vi "BlingLoop.vi"(5 "Cancel Ref":refnum<notifier>, 10 "Camera Ring Color":refnum<vi>, 11 "Target":string="10.24.68.5") -> (0 "error out":errorcluster)   [LabVIEW 2018]
uses:
  LedControlStates.ctl
  BlingLibrary/ControlState.ctl
  BlingLibrary/ConnectionType.ctl
  BlingLibrary/UdpConnection.ctl
  BlingLibrary/ChainState.ctl
  <vilib>/Platform/TimedLoop/XDataNode/timing_clust.ctl
  <vilib>/Platform/TimedLoop/XDataNode/nitl_modes.ctl
  <vilib>/Platform/TimedLoop/XDataNode/wakeup.ctl
  <vilib>/Rock Robotics/Network Tables/NT Read Number.vi
  <vilib>/Rock Robotics/Network Tables/NT Read Boolean.vi
  <vilib>/Rock Robotics/Network Tables/NT Read Raw.vi
  <vilib>/Platform/TimedLoop/XDataNode/XDataNode.xnode
  <vilib>/Platform/TimedLoop/XDataNode/XDNodeRunTimeDep.lvlib
  BlingLibrary/ArduinoSerialBling.lvlib
panel:
  in  "Mode":T1=enum."Ethernet"
  out "COM Overhead":i64 format="%.0f ms"
  in  "Get State":bool
  out "State":string
  in  "NT Offline Mode":bool
  in  "Offline Driver Color":u32(colorbox)
  in  "Offline Lift":dbl(slide) scale=0.0..100.0
  in  "Offline State":T2
  out "ControlState out":T3 {"ChainMask" format="0x%02x"}
  out "Bling State":T2
  out "LEDs":u32[](array[colorbox])
  in  "Manual Stop":bool
  # "Debug Controls"
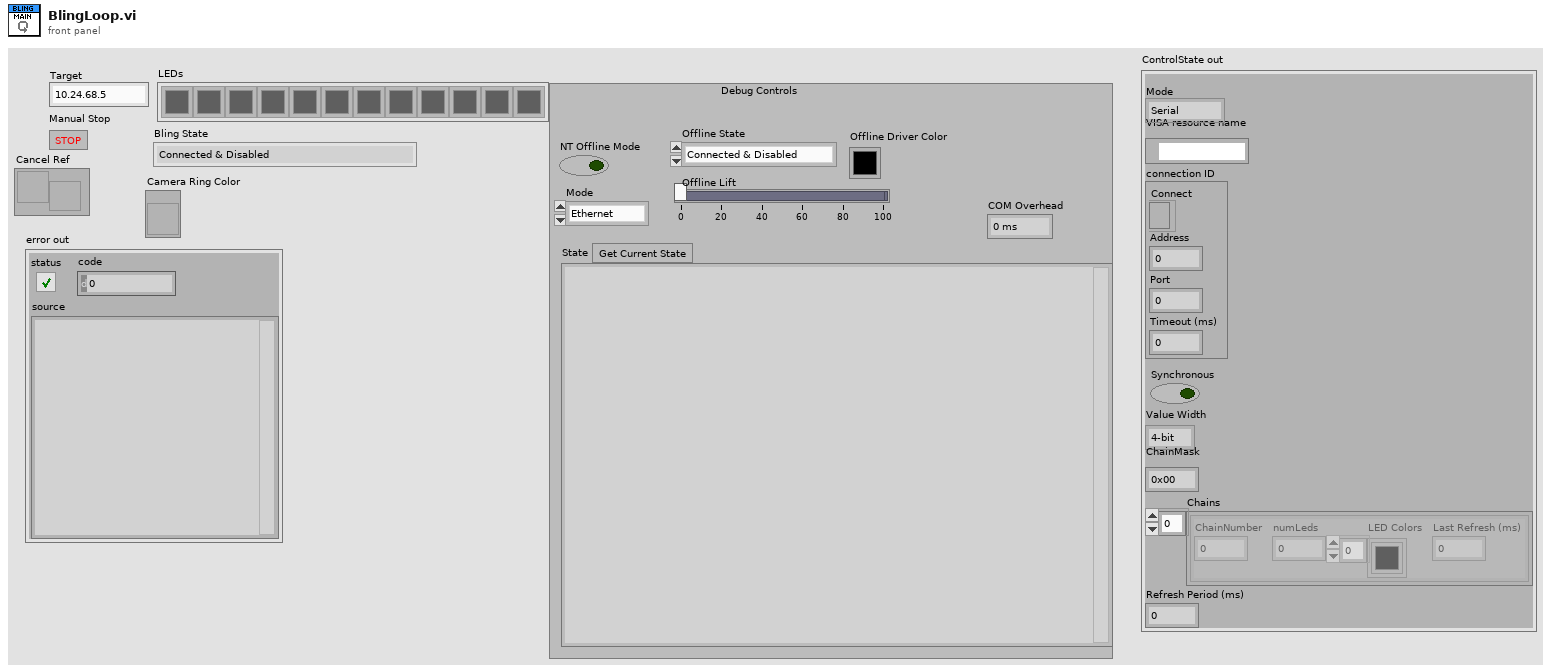
[diagram p1: front panel]
types:
  T1 = typedef "ConnectionType.ctl" = enum16{"Serial", "Ethernet", "Offline"}
  T2 = typedef "LedControlStates.ctl" = enum16{"Connected & Disabled", "Disconnected from RoboRIO", "Brownout", "Low Pressure", "Have Hatch", "Have Cargo", "ADAS Ready", "ADAS Active", "Lift Active", "Shutting Down", "Driving", "Driver Color"}
  T3 = typedef "ArduinoSerialBling.lvlib/ControlState.ctl" = cluster{"Mode":T1, "VISA resource name":refnum<visa-resource-name>, "connection ID":T4, "Synchronous":bool, "Value Width":enum16{"4-bit", "8-bit"}, "ChainMask":u8, "Chains":T5[], "Refresh Period (ms)":u32}
  T4 = typedef "UdpConnection.ctl" = cluster{"Connect":refnum<k16>, "Address":u32, "Port":u16, "Timeout (ms)":i32}
  T5 = typedef "ArduinoSerialBling.lvlib/ChainState.ctl" = cluster{"ChainNumber":u8, "numLeds":u8, "LED Colors":u32[], "Last Refresh (ms)":u32}
  T6 = typedef "XDNodeRunTimeDep.lvlib/timing_clust.ctl" = cluster{"Expected End [f-1]":u64, "Actual End [f-1]":u64, "Finished Late? [f-1]":bool, "Expected End [i-1]":u64, "Actual End [i-1]":u64, "Finished Late? [i-1]":bool, "Expected Start [i]":u64, "Actual Start [i]":u64, "Expected Start [f]":u64, "Actual Start [f]":u64, "Source Name":string, "Structure Name":string, "Period":i64, "Deadline":i64, "Offset":i64, "Start":i64, "Priority":i32, "Timeout":i32, "Mode":T7, "Wakeup Reason":T8, "Error":errorcluster, "Source Type":string, "Secondary Source Type":string, "Global End Time":u64, "Global Start Time":u64, "Frame Duration":u64, "Iteration Duration":u64, "Assigned CPU":i32, "I/O Scan Engine Mode":u32}
  T7 = typedef "XDNodeRunTimeDep.lvlib/nitl_modes.ctl" = enum32{"No Change", "Process missed periods, maintain original phase", "Discard missed periods, maintain original phase", "Process missed periods, ignore original phase", "Discard missed periods, ignore original phase"}
  T8 = typedef "XDNodeRunTimeDep.lvlib/wakeup.ctl" = enum32{"Normal", "Aborted", "Asynchronous wakeup", "Timing source error", "Timed loop error", "Timeout"}
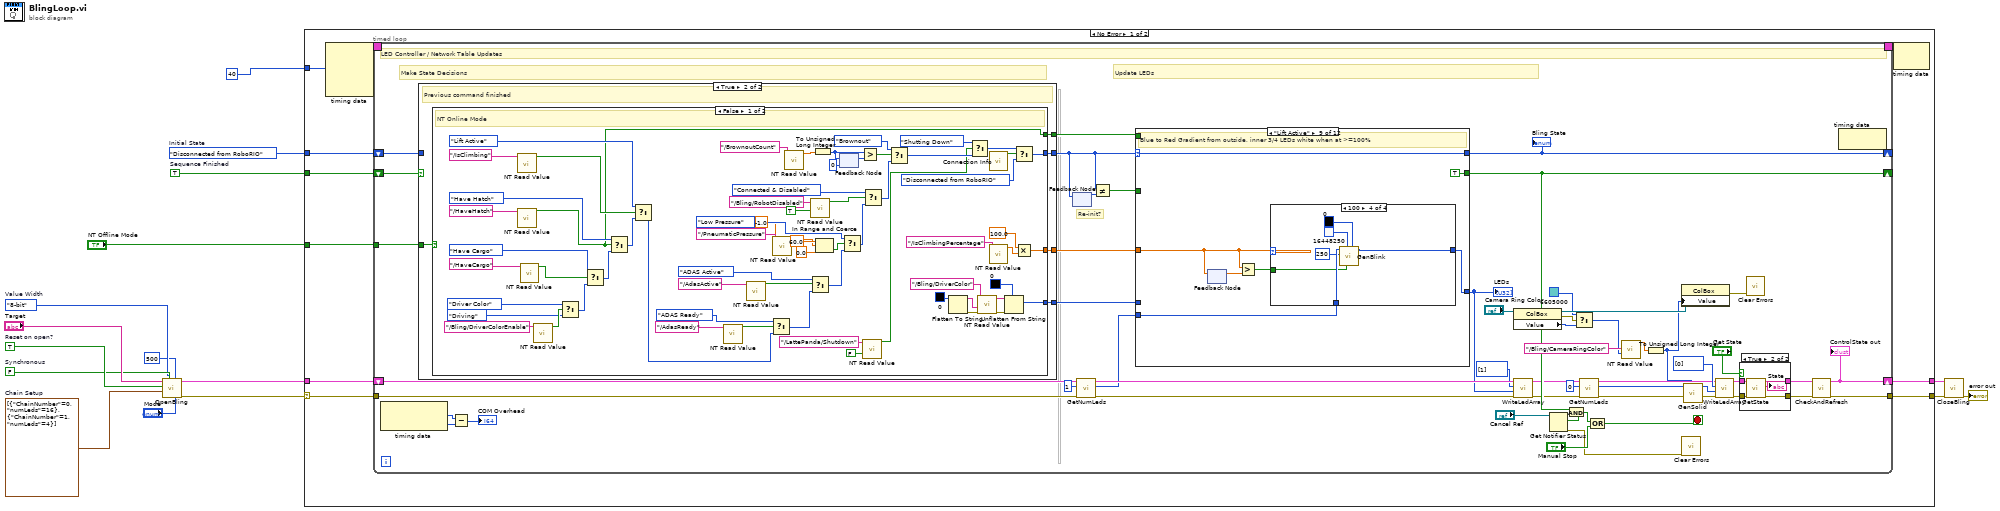
[diagram p0: block diagram]
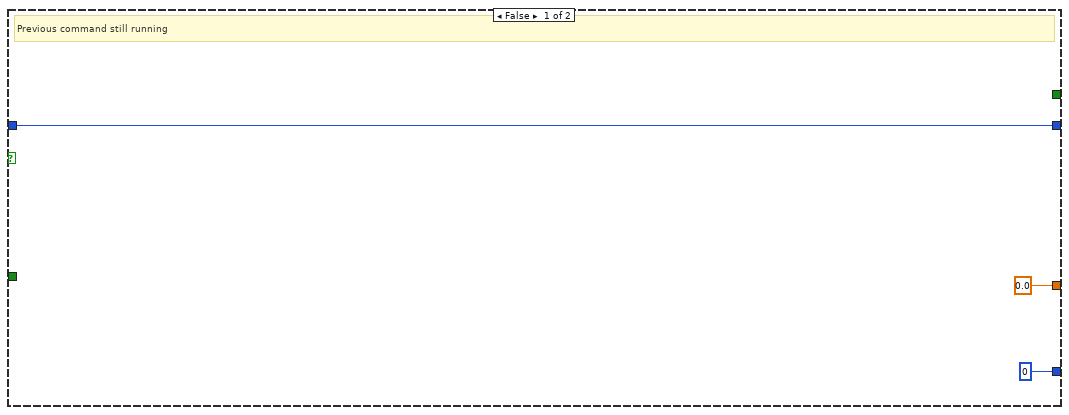
[diagram p3: hidden frame]
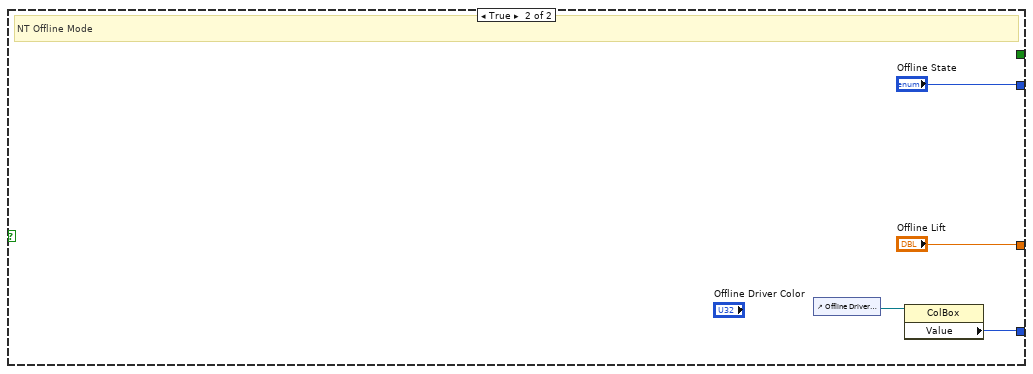
[diagram p4: hidden frame]
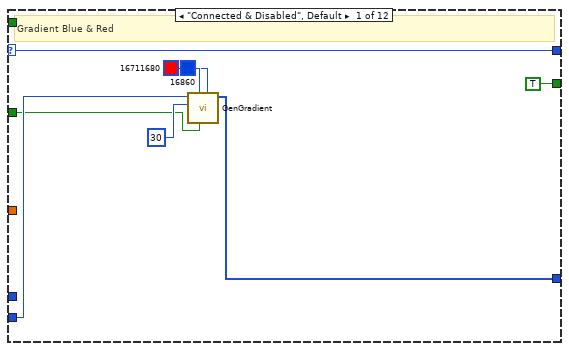
[diagram p5: hidden frame]
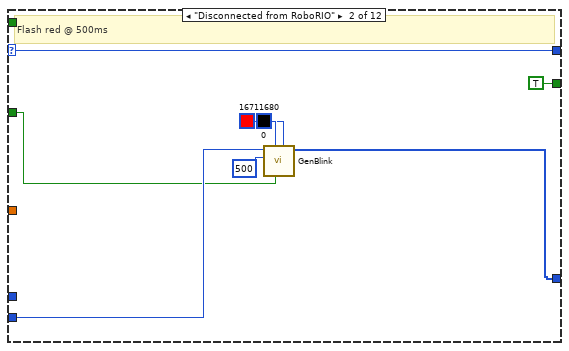
[diagram p6: hidden frame]
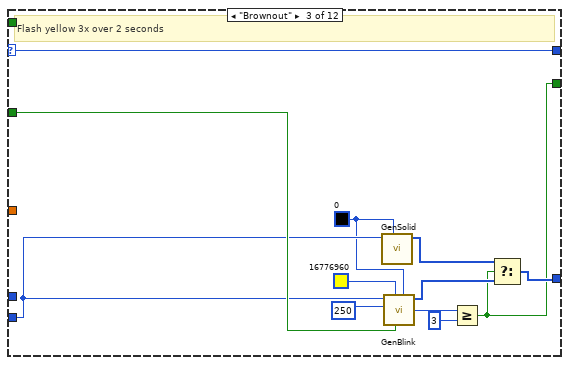
[diagram p7: hidden frame]
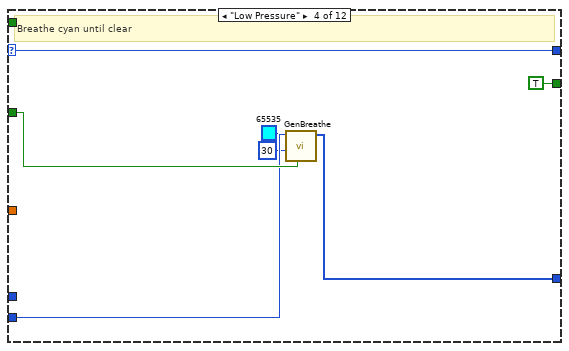
[diagram p8: hidden frame]
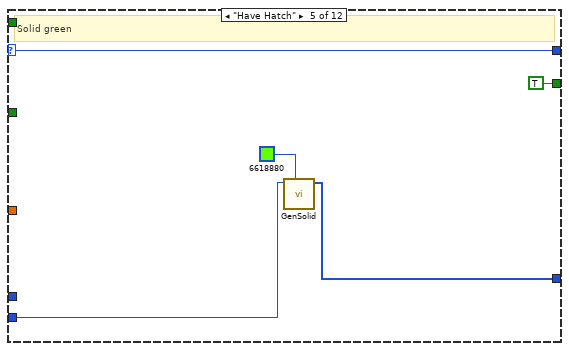
[diagram p9: hidden frame]
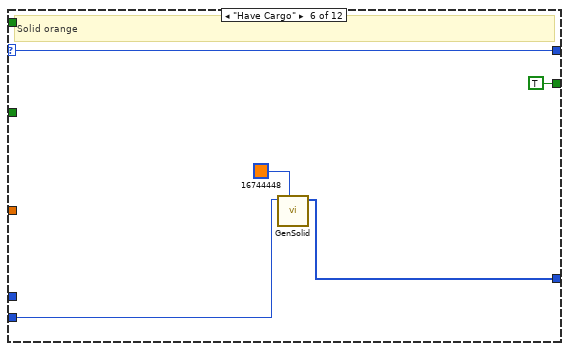
[diagram p10: hidden frame]
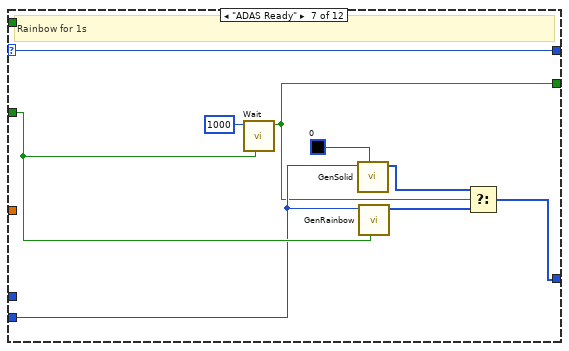
[diagram p11: hidden frame]
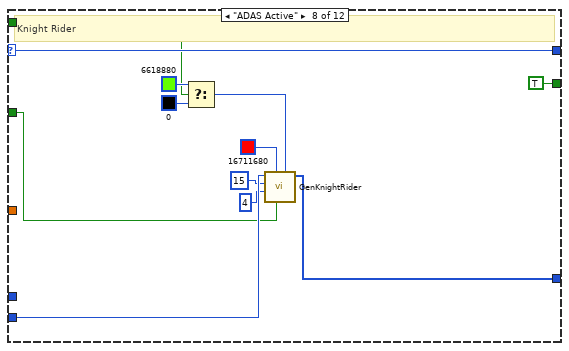
[diagram p12: hidden frame]
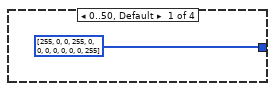
[diagram p13: hidden frame]
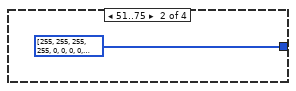
[diagram p14: hidden frame]
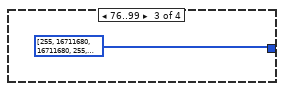
[diagram p15: hidden frame]
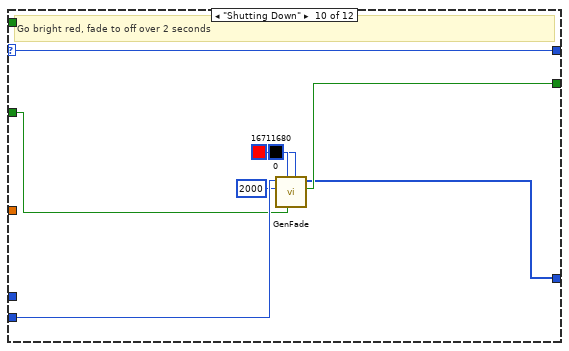
[diagram p16: hidden frame]
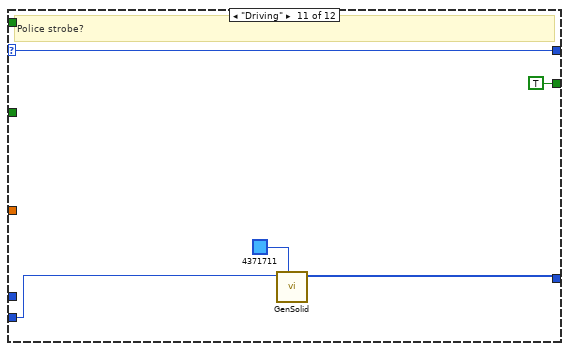
[diagram p17: hidden frame]
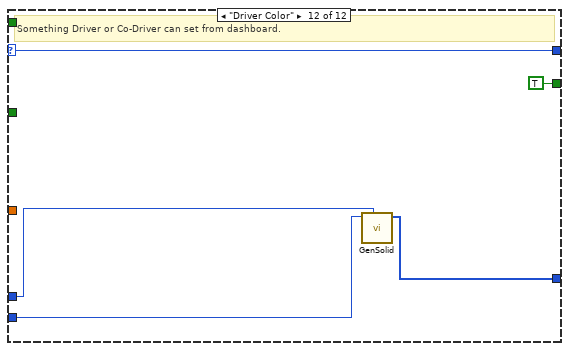
[diagram p18: hidden frame]
diagram:
  w7 = TRUE  # Sequence Finished
  w8 = LedControlStates."Disconnected from RoboRIO"  # Initial State
  w11 = enum16{"4-bit", "8-bit"}."8-bit"  # Value Width
  w12 = FALSE  # Synchronous
  w13 = cluster{"ChainNumber":u8, "numLeds":u8}[] [{"ChainNumber"=0, "numLeds"=16}, {"ChainNumber"=1, "numLeds"=4}]  # Chain Setup
  w14 = TRUE  # Reset on open?
  n1 = call "OpenBling.vi"("Mode"="Mode", "Refresh Period (ms)"=u32 500, "Synchronous"=w12, "Value Width"=w11, "Chain Setup"=w13, "Reset on open?"=w14, "Address/COM Port"="Target") -> ("error out"=w3:errorcluster, "ControlState"=w1:T3)  [unwired: 3 in]
  n2 = case shown="No Error" w3 {
    selector: w3 -> [w17 w273]
    tunnel: i64 40 ("Period") -> [w24 _]
    tunnel: [w23 w273] -> w10
    tunnel: [w22 w274] -> w9
    tunnel: w8 -> [w21 _]
    tunnel: w7 -> [w20 _]
    tunnel: "NT Offline Mode" -> [w19 _]
    tunnel: w1 -> [w18 w274]
    frame No Error {
      n3 = node-c288(w24) -> (w26:T6)  [unwired: 3 in]
      n4 = timed-loop {
        timing: w26 -> [_]
        timing-out: [_] -> w25
        tunnel: w17 -> [w72]
        tunnel: [w52] -> w23
        shift-right: [w78] -> _
        shift-left: w21 -> [w76]
        shift-right: [w59] -> _
        shift-left: w20 -> [w77]
        tunnel: w19 -> [w66]
        shift-right: [w51] -> w22
        shift-left: w18 -> [w28]
        stop <- w79 stop-if-true
        # "Re-init?"
        # "Update LEDs"
        # "Make State Decisions"
        # "LED Controller / Network Table Updates"
        n5 = node-c288() -> (w63:i64, w62:i64)  [unwired: 1 in]
        n6 = case shown="True" w77 {
          tunnel: [w89 w94] -> w74
          tunnel: w76 -> [w89 _]
          tunnel: [0.0 w93] -> w68
          tunnel: [u32 0 w92] -> w67
          tunnel: w66 -> [_ w91]
          tunnel: [_ w90] -> w27
          frame False {
            # "Previous command still running"
          }
          frame True {
            # "Previous command finished"
            n7 = case shown="False" w91 {
              tunnel: [w158 "Offline State"] -> w94
              tunnel: [w113 "Offline Lift"] -> w93
              tunnel: [w105 w161] -> w92
              tunnel: [w95 _] -> w90
              frame False {
                # "NT Online Mode"
                n8 = call-poly <vilib>:"NT Read Value.vi"("Name"="/IsClimbing") -> ("Boolean"=w121:bool)  [unwired: 9 in, 1 out]
                n9 = call-poly <vilib>:"NT Read Value.vi"("Name"="/HaveHatch") -> ("Boolean"=w95:bool)  [unwired: 9 in, 1 out]
                n10 = call-poly <vilib>:"NT Read Value.vi"("Name"="/HaveCargo") -> ("Boolean"=w120:bool)  [unwired: 9 in, 1 out]
                n11 = call-poly <vilib>:"NT Read Value.vi"("Name"="/Bling/DriverColorEnable") -> ("Boolean"=w131:bool)  [unwired: 9 in, 1 out]
                n12 = Select(t=LedControlStates."Driver Color" ("BlingStates"), s=w131, f=LedControlStates."Driving" ("BlingStates")) -> (s? t:f=w128:T2)
                n13 = Select(t=LedControlStates."Have Cargo" ("BlingStates"), s=w120, f=w128) -> (s? t:f=w127:T2)
                n14 = Select(t=LedControlStates."Have Hatch" ("BlingStates"), s=w95, f=w127) -> (s? t:f=w126:T2)
                n15 = Select(t=LedControlStates."Lift Active" ("BlingStates"), s=w121, f=w126) -> (s? t:f=w125:T2)
                n16 = call-poly <vilib>:"NT Read Value.vi"("Name"="/AdasReady") -> ("Boolean"=w138:bool)  [unwired: 9 in, 1 out]
                n17 = call-poly <vilib>:"NT Read Value.vi"("Name"="/AdasActive") -> ("Boolean"=w139:bool)  [unwired: 9 in, 1 out]
                n18 = Select(t=LedControlStates."ADAS Ready" ("BlingStates"), s=w138, f=w125) -> (s? t:f=w135:T2)
                n19 = call-poly <vilib>:"NT Read Value.vi"("Default Value"=-1.0, "Name"="/PneumaticPressure") -> ("Numeric"=w99:dbl)  [unwired: 8 in, 1 out]
                n20 = call-poly <vilib>:"NT Read Value.vi"("Name"="/BrownoutCount") -> ("Numeric"=w155:dbl)  [unwired: 9 in, 1 out]
                n21 = call-poly <vilib>:"NT Read Value.vi"("Default Value"=TRUE, "Name"="/Bling/RobotDisabled") -> ("Boolean"=w140:bool)  [unwired: 8 in, 1 out]
                n22 = Select(t=LedControlStates."ADAS Active" ("BlingStates"), s=w139, f=w135) -> (s? t:f=w134:T2)
                n23 = To Unsigned Long Integer(number=w155) -> (unsigned 32bit integer=w153:u32)
                n24 = In Range and Coerce(upper limit=60.0, x=w99, lower limit=0.0) -> (In Range?=w97:bool)  [unwired: 1 out]
                n25 = feedback #1(u32 0) -> (w154:u32)
                n26 = feedback-in #1(w153) -> ()
                n27 = Select(t=LedControlStates."Low Pressure" ("BlingStates"), s=w97, f=w134) -> (s? t:f=w132:T2)
                n28 = Greater?(x=w153, y=w154) -> (0:w145:bool)
                n29 = call-poly <vilib>:"NT Read Value.vi"("Default Value"=FALSE ("Boolean"), "Name"="/LattePanda/Shutdown") -> ("Boolean"=w102:bool)  [unwired: 8 in, 1 out]
                n30 = Select(t=LedControlStates."Connected & Disabled" ("BlingStates"), s=w140, f=w132) -> (s? t:f=w141:T2)
                n31 = Select(t=LedControlStates."Brownout" ("BlingStates"), s=w145, f=w141) -> (s? t:f=w143:T2)
                n32 = Flatten To String(anything=u32 0) -> (data string=w111:string, error out=w110:errorcluster)  [unwired: 3 in, 1 out]
                n33 = Select(t=LedControlStates."Shutting Down" ("BlingStates"), s=w102, f=w143) -> (s? t:f=w147:T2)
                n34 = call-poly <vilib>:"NT Read Value.vi"("error in"=w110, "Default Value"=w111, "Name"="/Bling/DriverColor") -> ("error out"=w107:errorcluster, "Raw"=w109:string)  [unwired: 7 in]
                n35 = call <vilib>:"Connection Info.vi"() -> ("Connected"=w160:bool)  [unwired: 10 in, 1 out]
                n36 = call-poly <vilib>:"NT Read Value.vi"("Name"="/IsClimbingPercentage") -> ("Numeric"=w116:dbl)  [unwired: 9 in, 1 out]
                n37 = Unflatten From String(type=u32 0, binary string=w109, error in (no error)=w107) -> (value=w105:u32)  [unwired: 2 in, 2 out]
                n38 = Select(t=w147, s=w160, f=LedControlStates."Disconnected from RoboRIO" ("BlingStates")) -> (s? t:f=w158:T2)
                n39 = Multiply(x=100.0 ("y"), y=w116) -> (x*y=w113:dbl)
              }
              frame True {
                # "NT Offline Mode"
                n40 = control-ref of="Offline Driver Color"() -> (w162:refnum<vi>)
                n41 = property class="ColBox"(reference=w162) -> ("Value"=w161:u32)  [unwired: 1 in, 2 out]
              }
            }
          }
        }
        n42 = Subtract(x=w63, y=w62) -> (x-y=→"COM Overhead":i64)
        n43 = feedback-in #2(w74) -> ()
        n44 = feedback #2() -> (w75:T2)  [unwired: 1 in]
        n45 = call "GetNumLeds.vi"("error in (no error)"=w72, "Chain"=1, "ControlState"=w28) -> ("error out"=w69:errorcluster, "NumLeds"=w50:i32, "ControlState 2"=w70:T3)  [unwired: 6 in]
        n46 = Not Equal?(x=w74, y=w75) -> (x != y?=w73:bool)
        n47 = case shown="\"Lift Active\"" w74 {
          selector: w74 -> [w171 w180 w187 w198 w203 w208 w218 w229 w237 w254 w258 w261]
          tunnel: [w171 w180 w187 w198 w203 w208 w218 w229 w237 w254 w258 w261] -> w78
          tunnel: [TRUE TRUE w181 TRUE TRUE TRUE w211 TRUE TRUE w251 TRUE TRUE] -> w59
          tunnel: w73 -> [w165 w173 w189 w197 _ _ w216 w223 _ w247 _ _]
          tunnel: w50 -> [w170 w174 w184 w196 w201 w205 w212 w228 w234 w253 w257 w263]
          tunnel: [w166 w178 w186 w193 w200 w206 w210 w224 w235 w250 w256 w262] -> w49
          tunnel: w68 -> [_ _ _ _ _ _ _ _ w232 _ _ _]
          tunnel: w67 -> [_ _ _ _ _ _ _ _ _ _ _ w260]
          tunnel: w27 -> [_ _ _ _ _ _ _ w219 _ _ _ _]
          frame "Connected & Disabled", Default {
            # "Gradient Blue & Red"
            n48 = call "GenGradient.vi"("Color 2"=u32 16860, "Reset"=w165, "Color 1"=u32 16711680, "Sine Rate"=30, "NumLeds"=w170) -> ("LED Array"=w166:u32[])  [unwired: 6 in]
          }
          frame "Disconnected from RoboRIO" {
            # "Flash red @ 500ms"
            n49 = call "GenBlink.vi"("Color 2"=u32 0, "Reset"=w173, "Color 1"=u32 16711680, "Period (ms)"=500, "NumLeds"=w174) -> ("Array"=w178:u32[])  [unwired: 5 in, 1 out]
          }
          frame "Brownout" {
            w183 = u32 0 ("Color 2")
            # "Flash yellow 3x over 2 seconds"
            n50 = call "GenSolid.vi"("Color"=w183, "NumLeds"=w184) -> ("Array"=w182:u32[])  [unwired: 9 in]
            n51 = call "GenBlink.vi"("Color 2"=w183, "Reset"=w189, "Color 1"=u32 16776960, "Period (ms)"=250, "NumLeds"=w184) -> ("Iterator"=w190:i32, "Array"=w185:u32[])  [unwired: 5 in]
            n52 = Greater Or Equal?(x=w190, y=3) -> (x >= y?=w181:bool)
            n53 = Select(t=w182, s=w181, f=w185) -> (s? t:f=w186:u32[])
          }
          frame "Low Pressure" {
            # "Breathe cyan until clear"
            n54 = call "GenBreathe.vi"("Reset"=w197, "Sine Rate"=30, "Color Box"=u32 65535, "NumLeds"=w196) -> ("Array"=w193:u32[])  [unwired: 6 in, 1 out]
          }
          frame "Have Hatch" {
            # "Solid green"
            n55 = call "GenSolid.vi"("Color"=u32 6618880, "NumLeds"=w201) -> ("Array"=w200:u32[])  [unwired: 9 in]
          }
          frame "Have Cargo" {
            # "Solid orange"
            n56 = call "GenSolid.vi"("Color"=u32 16744448, "NumLeds"=w205) -> ("Array"=w206:u32[])  [unwired: 9 in]
          }
          frame "ADAS Ready" {
            # "Rainbow for 1s"
            n57 = call "Wait.vi"("Reset"=w216, "milliseconds to wait"=1000) -> ("Finished"=w211:bool)  [unwired: 9 in]
            n58 = call "GenSolid.vi"("Color"=u32 0 ("Color 2"), "NumLeds"=w212) -> ("Array"=w214:u32[])  [unwired: 9 in]
            n59 = call "GenRainbow.vi"("Reset"=w216, "NumLeds"=w212) -> ("Rainbow"=w213:u32[])  [unwired: 9 in]
            n60 = Select(t=w214, s=w211, f=w213) -> (s? t:f=w210:u32[])
          }
          frame "ADAS Active" {
            # "Knight Rider"
            n61 = Select(t=u32 6618880 ("Color"), s=w219, f=u32 0 ("Background Color")) -> (s? t:f=w220:u32)
            n62 = call "GenKnightRider.vi"("Background Color"=w220, "Reset"=w223, "Foreground Color"=u32 16711680, "Blending LEDs"=u8 4, "Sine Rate"=15, "NumLeds"=w228) -> ("Array"=w224:u32[])  [unwired: 4 in, 1 out]
          }
          frame "Lift Active" {
            # "Blue to Red Gradient from outside, inner 3/4 LEDs white when at >=100%"
            n63 = feedback-in #3(w232) -> ()
            n64 = feedback #3() -> (w233:dbl)  [unwired: 1 in]
            n65 = Greater?(x=w232, y=w233) -> (0:w231:bool)
            n66 = case shown="100" w232 {
              tunnel: [u32[] [255, 0, 0, 255, 0, 0, 0, 0, 0, 0, 0, 255] u32[] [255, 255, 255, 255, 0, 0, 0, 0, 16711680, 255, 255, 255] u32[] [255, 16711680, 16711680, 255, 16711680, 0, 0, 16711680, 16711680, 255, 255, 255] w241] -> w235
              tunnel: w234 -> [_ _ _ w246]
              tunnel: w231 -> [_ _ _ w242]
              frame 0..50, Default {
              }
              frame 51..75 {
              }
              frame 76..99 {
              }
              frame 100 {
                n67 = call "GenBlink.vi"("Color 2"=u32 0, "Reset"=w242, "Color 1"=u32 16448250, "Period (ms)"=250, "NumLeds"=w246) -> ("Array"=w241:u32[])  [unwired: 5 in, 1 out]
              }
            }
          }
          frame "Shutting Down" {
            # "Go bright red, fade to off over 2 seconds"
            n68 = call "GenFade.vi"("End Color"=u32 0, "Reset"=w247, "Start Color"=u32 16711680, "Total Time (ms)"=u32 2000, "NumLeds"=w253) -> ("Finished"=w251:bool, "Array"=w250:u32[])  [unwired: 5 in]
          }
          frame "Driving" {
            # "Police strobe?"
            n69 = call "GenSolid.vi"("Color"=u32 4371711, "NumLeds"=w257) -> ("Array"=w256:u32[])  [unwired: 9 in]
          }
          frame "Driver Color" {
            # "Something Driver or Co-Driver can set from dashboard."
            n70 = call "GenSolid.vi"("Color"=w260, "NumLeds"=w263) -> ("Array"=w262:u32[])  [unwired: 9 in]
          }
        }
        "LEDs" <- w49
        "Bling State" <- w78
        n71 = property class="ColBox"(reference="Camera Ring Color") -> (reference out=w35:refnum<vi>, error out=w32:errorcluster, "Value"=w31:u32)  [unwired: 1 in]
        n72 = call "WriteLedArray.vi"("error in (no error)"=w69, "LED Colors"=w49, "Chains"=u8[] [1], "ControlState in"=w70) -> ("error out"=w41:errorcluster, "ControlState out"=w42:T3)  [unwired: 5 in, 1 out]
        n73 = Get Notifier Status(notifier="Cancel Ref") -> (current notification=w60:bool, error out=w55:errorcluster)  [unwired: 1 in, 3 out]
        n74 = And(x=w59, y=w60) -> (x .and. y?=w58:bool)
        n75 = Select(t=u32 6605000 ("Color"), s=w32, f=w31) -> (s? t:f=w30:u32)
        n76 = call "GetNumLeds.vi"("error in (no error)"=w41, "Chain"=0, "ControlState"=w42) -> ("error out"=w44:errorcluster, "NumLeds"=w46:i32, "ControlState 2"=w45:T3)  [unwired: 6 in]
        n77 = Compound Arithmetic op=OR(w58, "Manual Stop") -> (w79:bool)
        n78 = call-poly <vilib>:"NT Read Value.vi"("Default Value"=w30, "Name"="/Bling/CameraRingColor") -> ("Numeric"=w37:dbl)  [unwired: 8 in, 1 out]
        n79 = To Unsigned Long Integer(number=w37) -> (unsigned 32bit integer=w33:u32)
        n80 = property class="ColBox"(reference=w35, "Value"=w33) -> (error out=w34:errorcluster)  [unwired: 1 in, 1 out]
        n81 = call <vilib>:"Clear Errors.vi"("error in (no error)"=w55) -> ()  [unwired: 5 in, 2 out]
        n82 = call "GenSolid.vi"("Color"=w33, "NumLeds"=w46) -> ("Array"=w43:u32[])  [unwired: 9 in]
        n83 = call "WriteLedArray.vi"("error in (no error)"=w44, "LED Colors"=w43, "Chains"=u8[] [0], "ControlState in"=w45) -> ("error out"=w39:errorcluster, "ControlState out"=w40:T3)  [unwired: 5 in, 1 out]
        n84 = case shown="True" "Get State" {
          tunnel: [w81 w86] -> w54
          tunnel: [w80 w85] -> w53
          tunnel: w40 -> [w81 w83]
          tunnel: w39 -> [w80 w82]
          frame False {
          }
          frame True {
            n85 = call "GetState.vi"("error in (no error)"=w82, "ControlState in"=w83) -> ("error out"=w85:errorcluster, "State"=→"State":string, "ControlState out"=w86:T3)  [unwired: 7 in]
          }
        }
        n86 = call <vilib>:"Clear Errors.vi"("error in (no error)"=w34) -> ()  [unwired: 5 in, 2 out]
        n87 = call "CheckAndRefresh.vi"("error in (no error)"=w53, "ControlState in"=w54) -> ("error out"=w52:errorcluster, "ControlState out"=w51:T3)  [unwired: 8 in]
        "ControlState out" <- w51
        n88 = node-c288() -> ()  [unwired: 1 in, 1 out]
      }
      n89 = node-c288(w25) -> ()  [unwired: 1 out]
    }
    frame Error {
    }
  }
  n90 = call "CloseBling.vi"("error in (no error)"=w10, "ControlState in"=w9) -> ("error out"=→"error out":errorcluster)  [unwired: 9 in]
